vi "main.vi"() -> ()   [LabVIEW 2014]
doc: "This is the Main VI that uses Producer/Consumer Structure to present the UI.\nit consists of 2 taps for normal and admin users.\nadmin tab/interface is hidden by default until admin is logged in."
uses:
  <vilib>/addons/database/_DB Variant To Data/Database Variant To Data.xnode
panel:
  out "Cashier":dbl format="%#_6f"
  out "Logged User":string
  in  "Tab Control":enum32{"operator", "Supervisor"}(tab)
  in  "stop":bool
  in  "Purchase":bool
  in  "Quantity":dbl min=0.0
  in  "Product":string(combo)
  in  "Paid":dbl min=0.0 format="%#_6f"
  out "Cost":dbl format="%#_6f"
  out "Change":dbl format="%#_6f"
  in  "change user":bool
  in  "file name":path=path "C:/vendingMC/history.xml"
  in  "Time To":timestamp format="%<%H:%M:%S\n%Y/%m/%d>T"
  in  "Time From":timestamp format="%<%H:%M:%S\n%Y/%m/%d>T"
  in  "Price":dbl min=0.0
  in  "Type":string(combo)="normal"
  in  "Add Quantity":dbl
  in  "Generate XML":bool
  in  "add product":bool
  in  "Add Name":string
  in  "Delete User":bool
  in  "Register":bool
  in  "Edit password":string
  in  "Edit username":string
  # "Vending Machine"
  # "Select Product to Buy"
  # "Register New User"
  # "Add/Update Product"
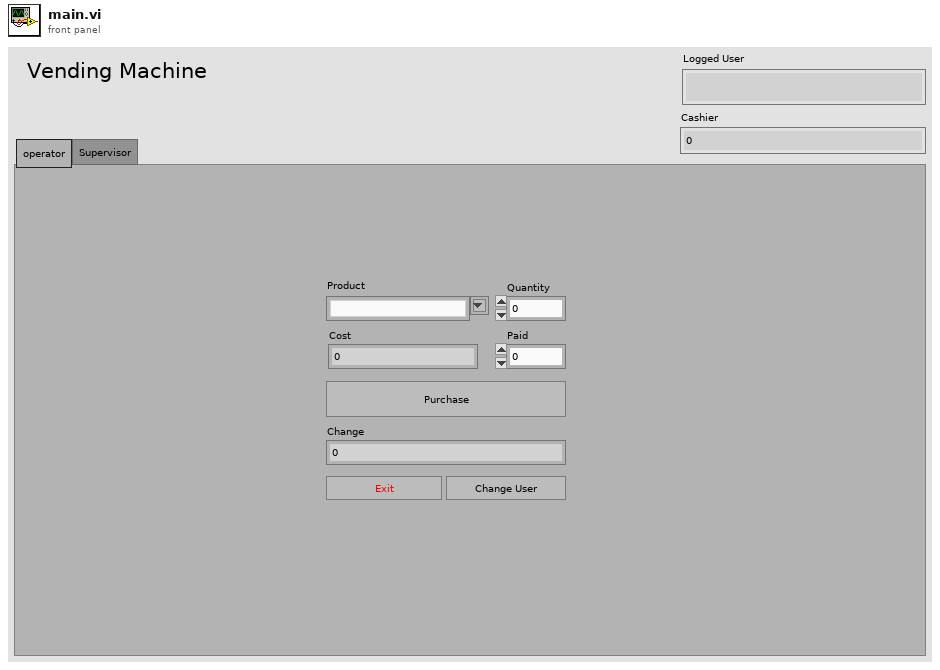
[diagram p1: front panel]
types:
  T1 = enum8{"Enabled", "Disabled", "Disabled and Grayed Out"}
  T2 = cluster{"date/time string":string, string, dbl, "Cost":dbl, dbl, dbl, "Logged User":string, "date/time string":string}
  T3 = enum16{"Left Button", "Center Button", "Right Button", "Window Close"}
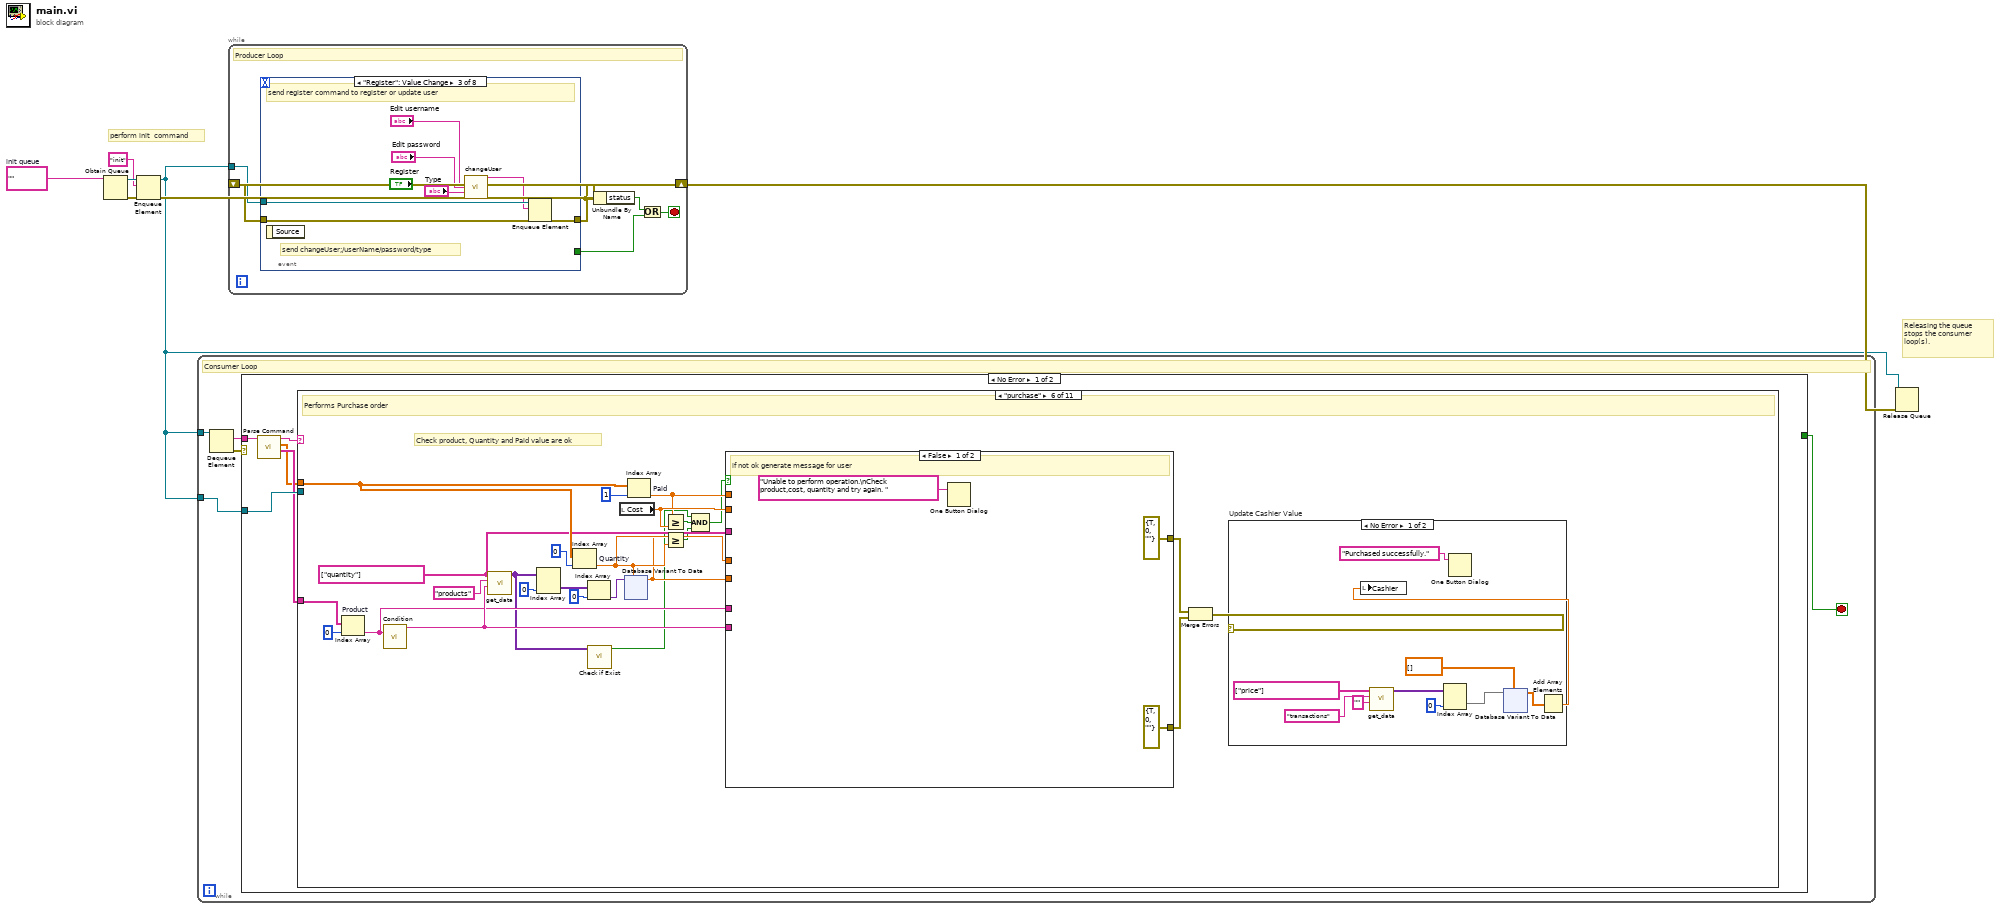
[diagram p0: block diagram]
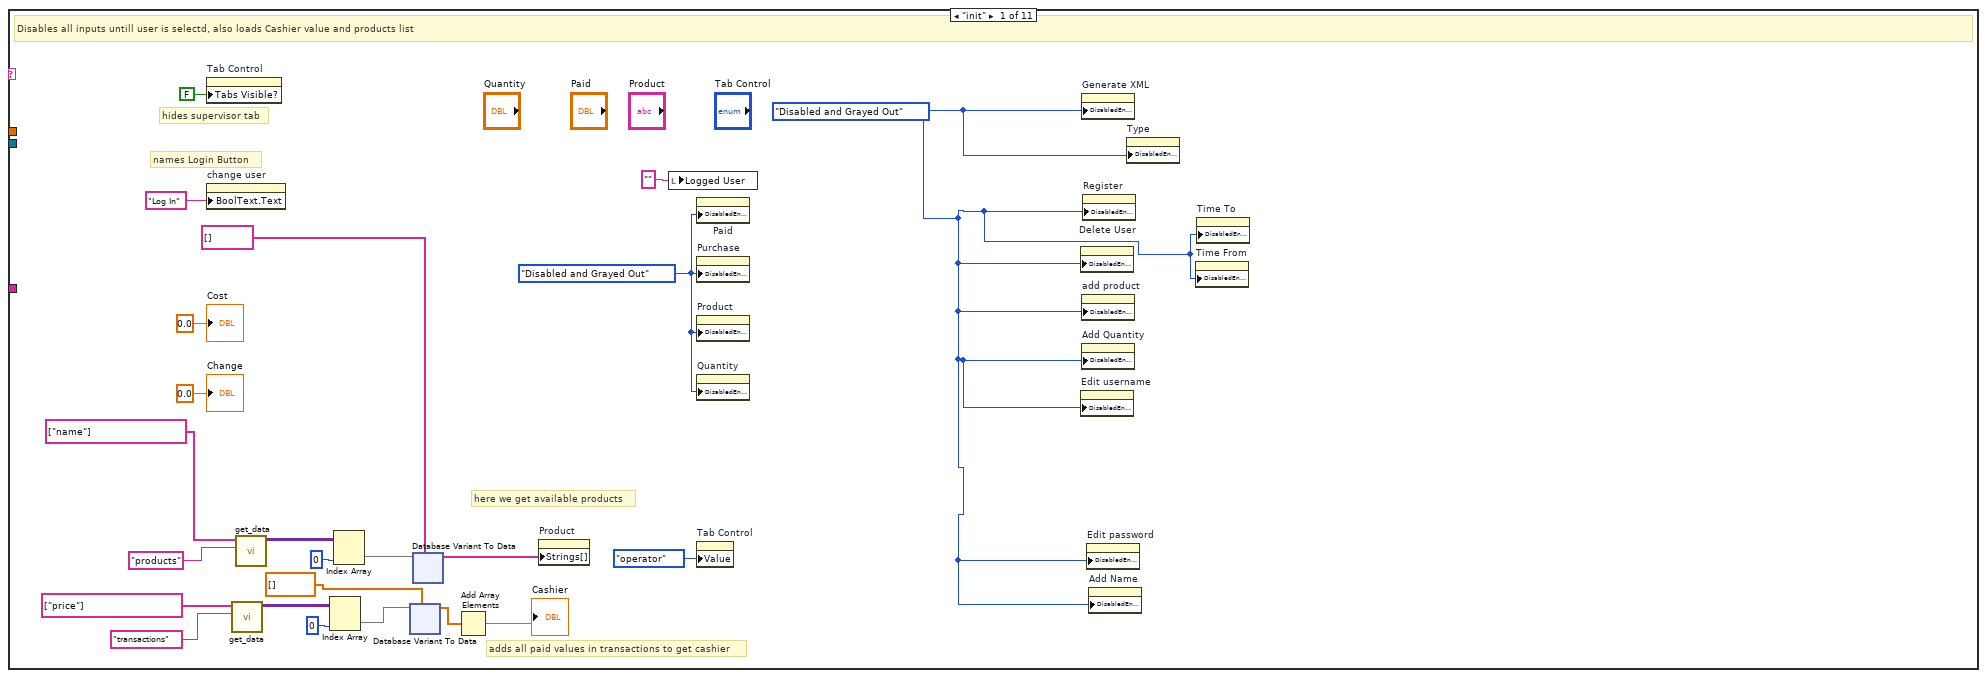
[diagram p2: hidden frame]
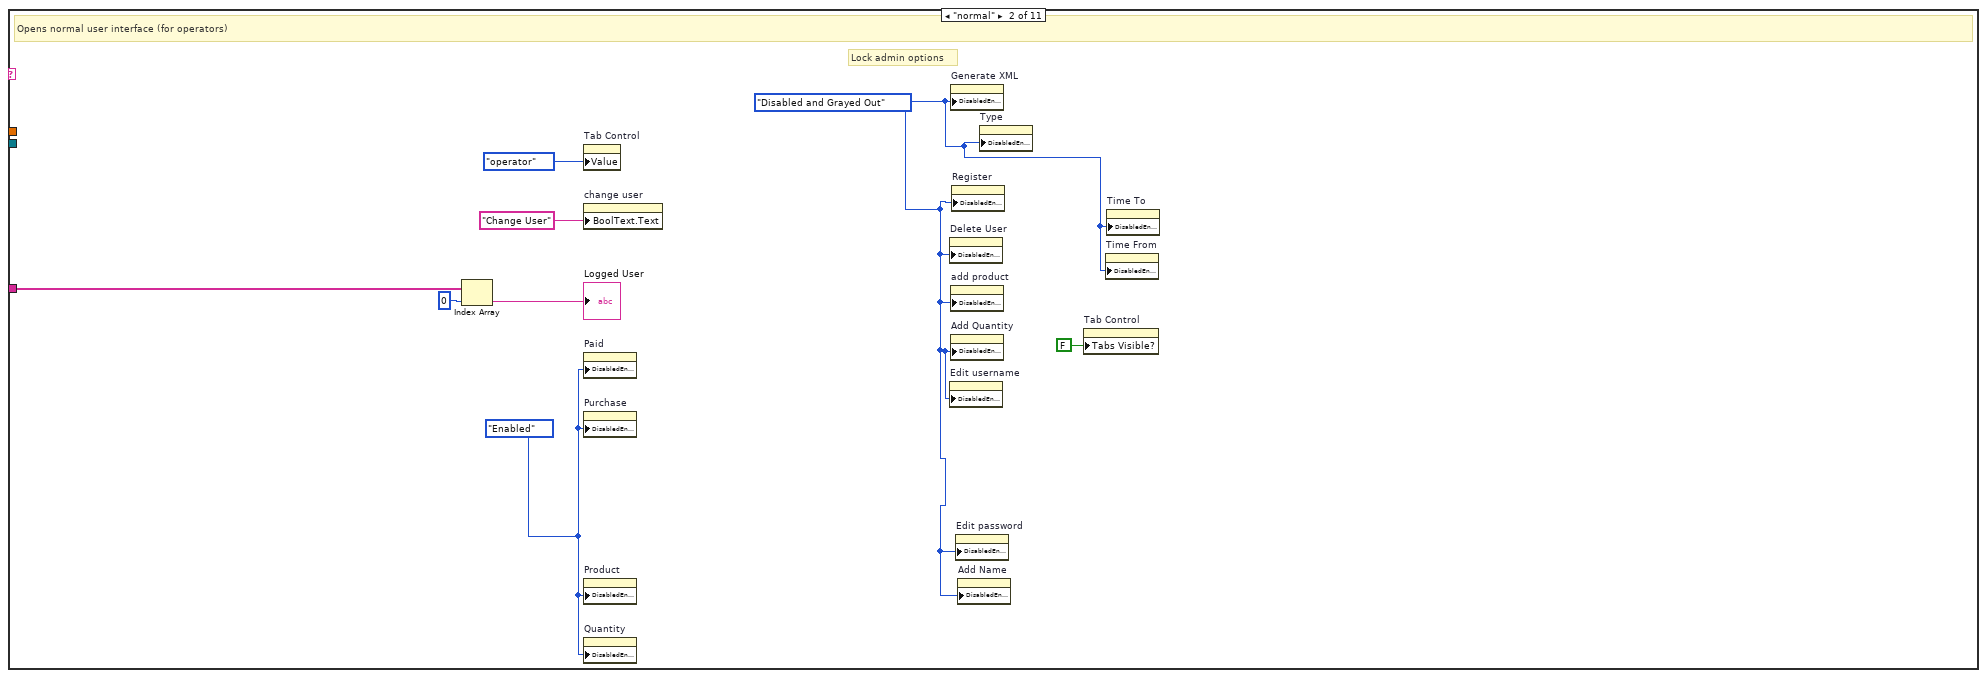
[diagram p3: hidden frame]
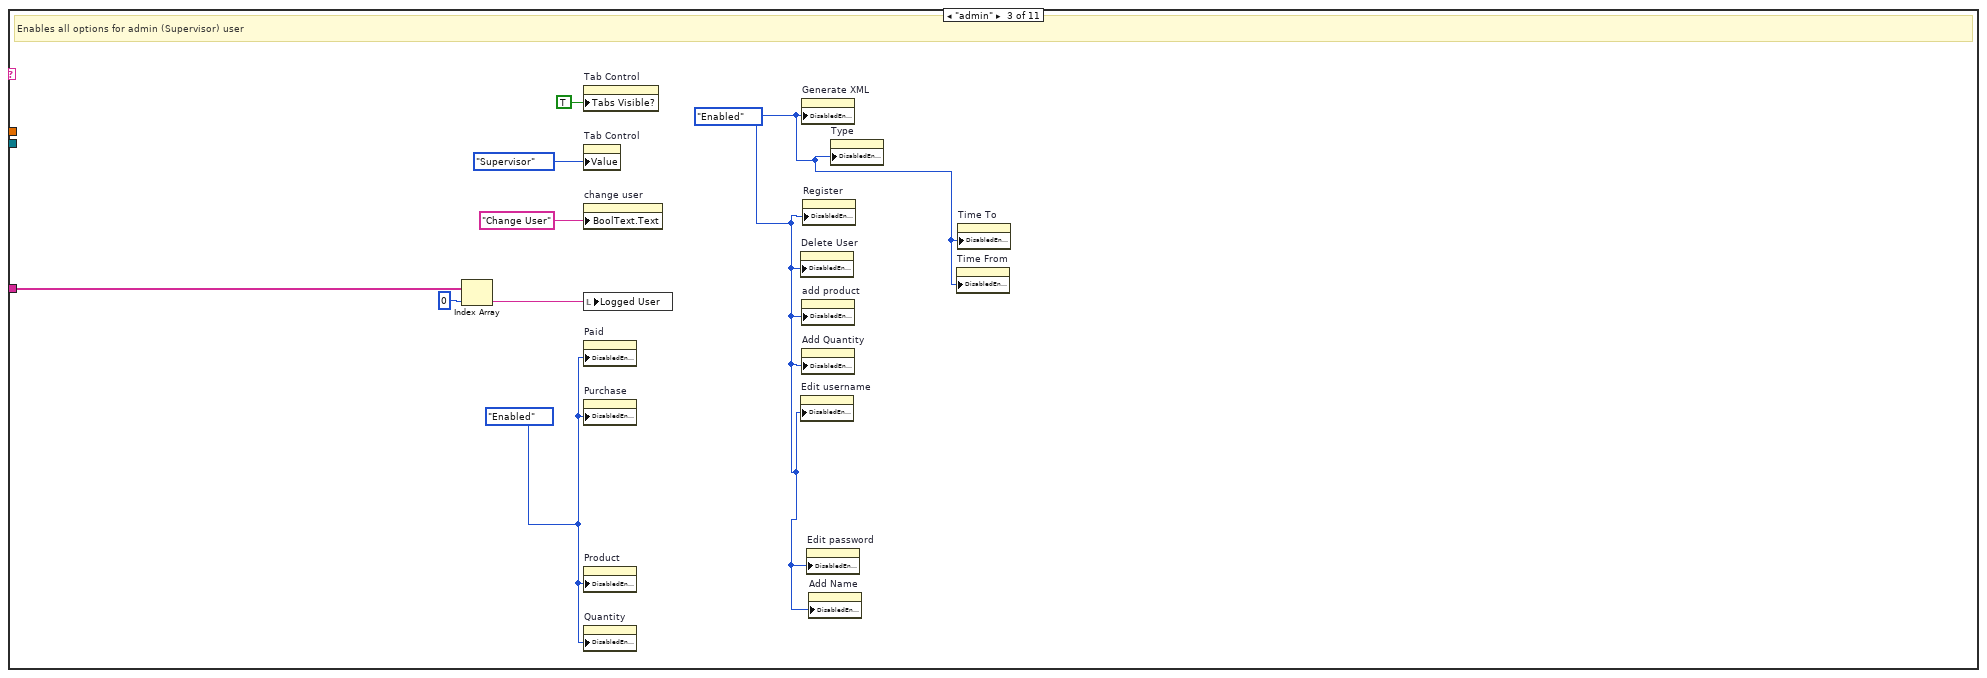
[diagram p4: hidden frame]
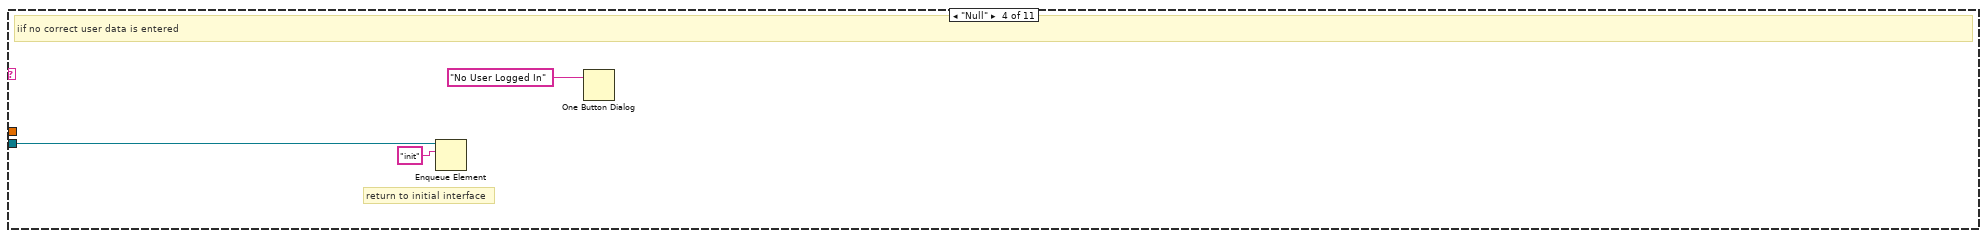
[diagram p5: hidden frame]
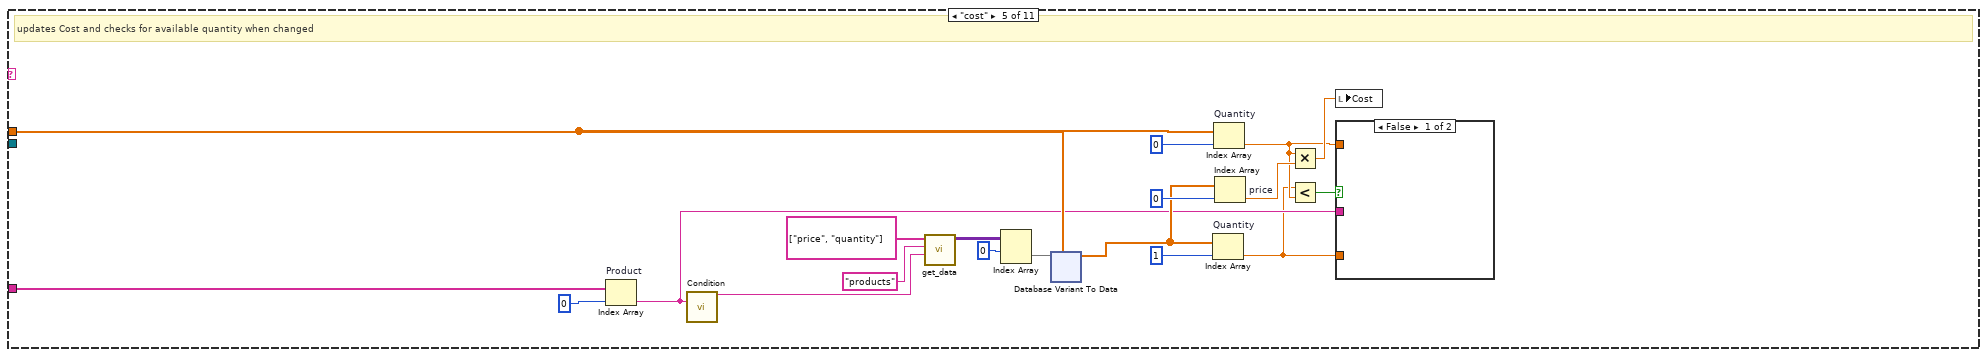
[diagram p6: hidden frame]
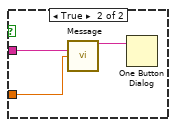
[diagram p7: hidden frame]
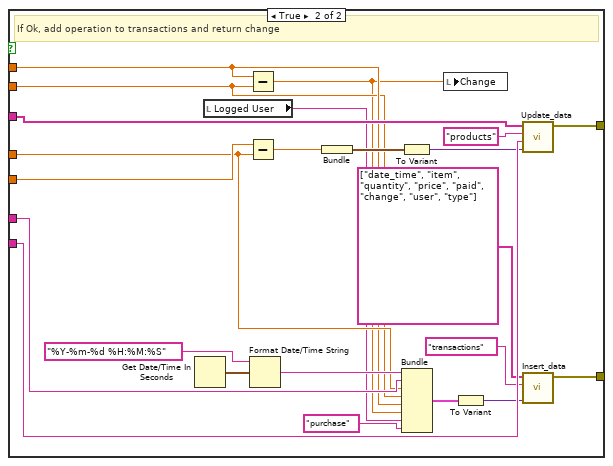
[diagram p9: hidden frame]
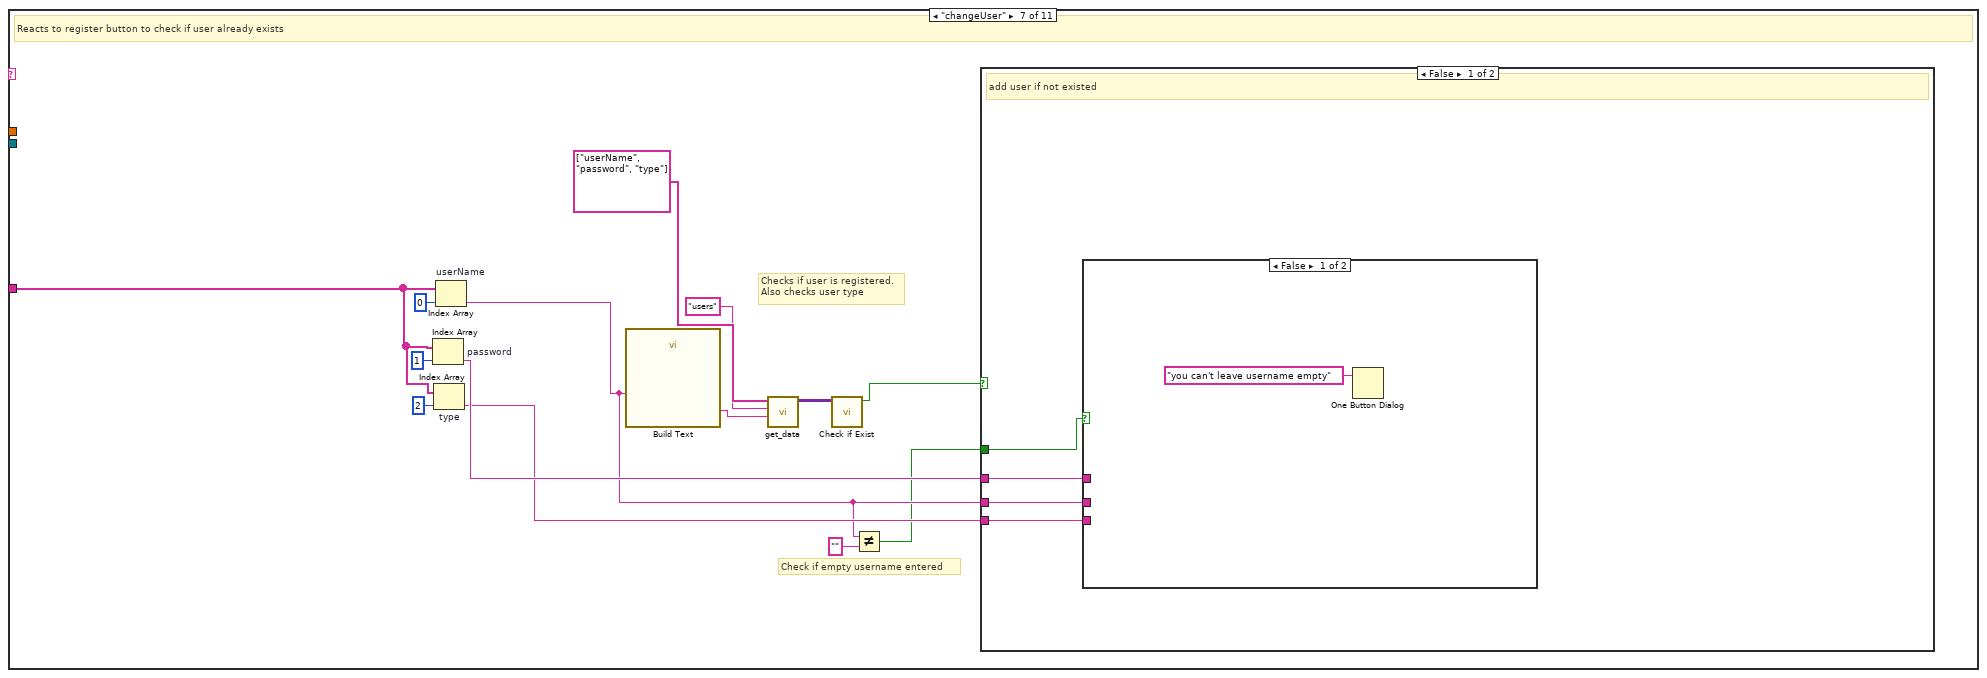
[diagram p10: hidden frame]
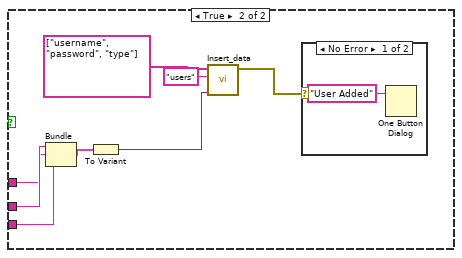
[diagram p11: hidden frame]
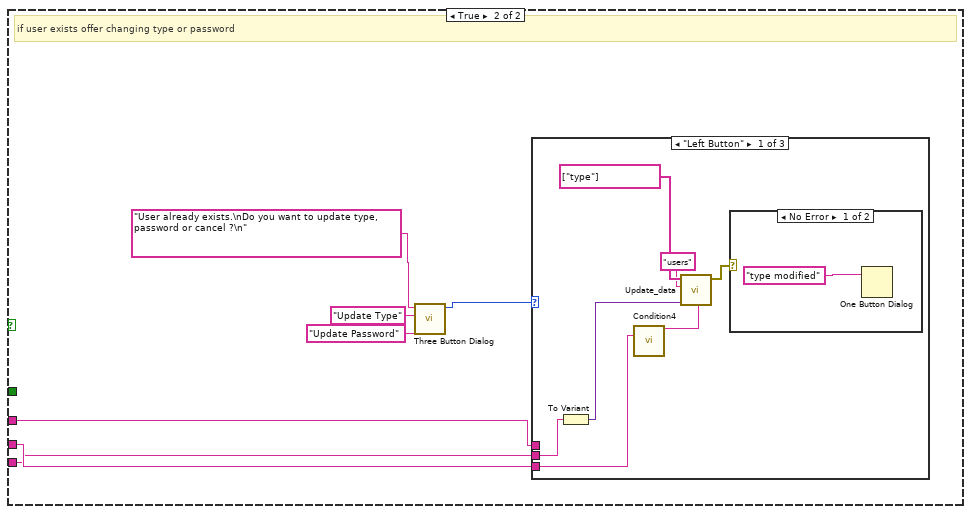
[diagram p13: hidden frame]
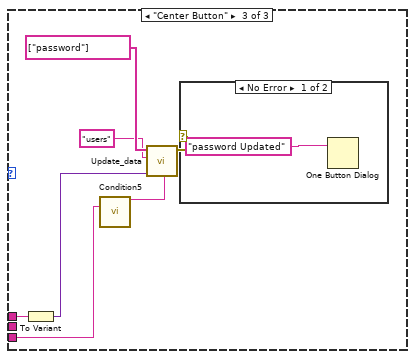
[diagram p16: hidden frame]
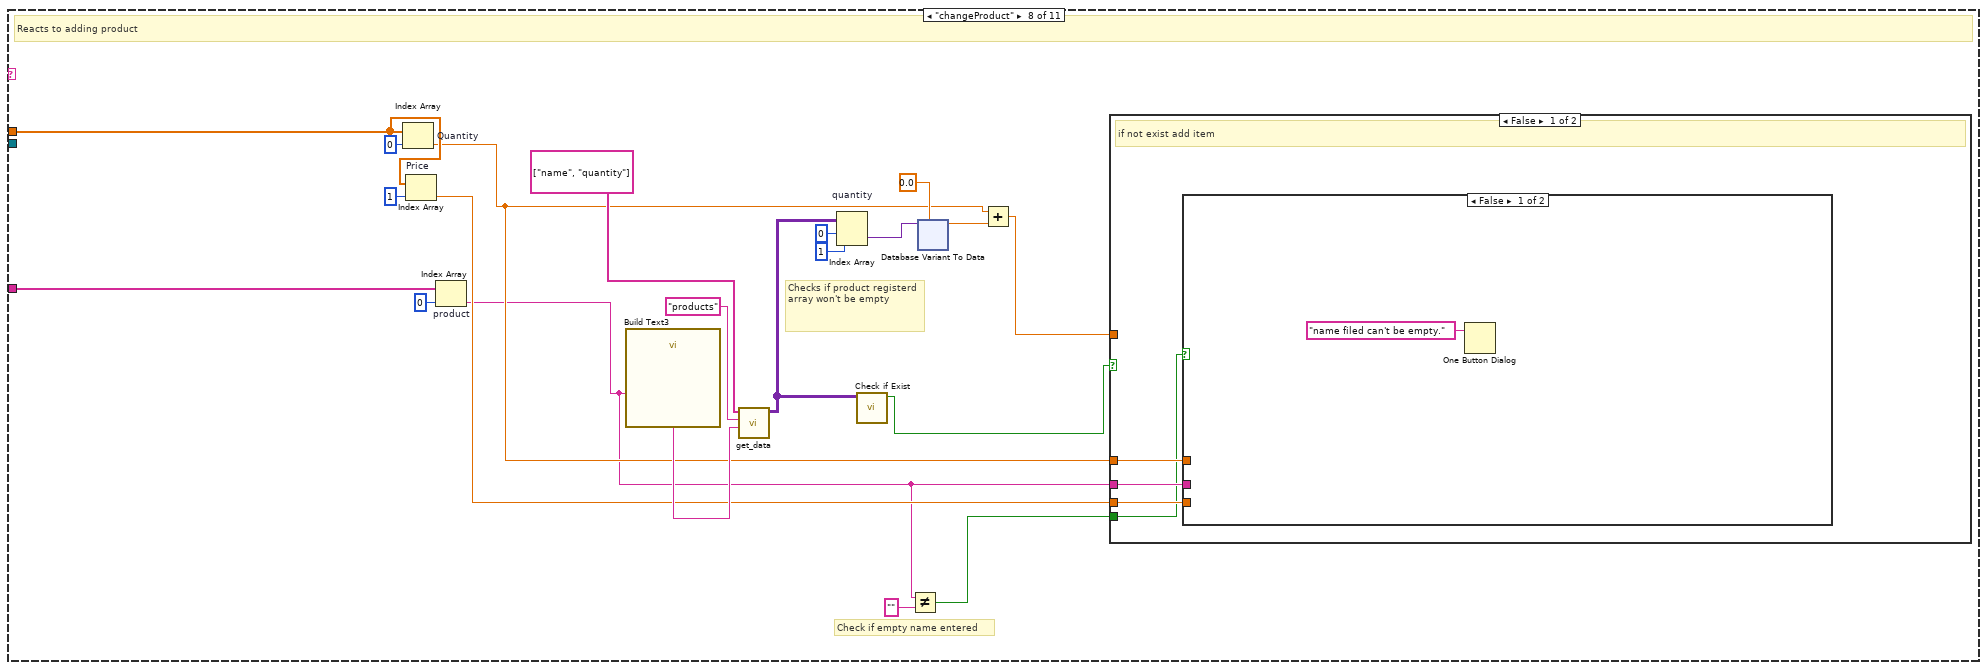
[diagram p18: hidden frame]
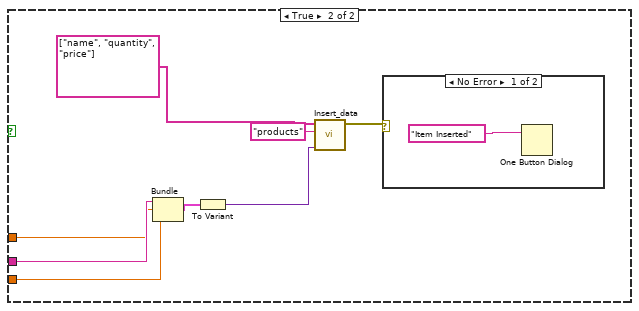
[diagram p19: hidden frame]
diagram:
  w6 = ""  # init queue
  # "perform init  command"
  # "Releasing the queue stops the consumer loop(s)."
  n1 = Obtain Queue(element data type=w6) -> (queue out=w5:refnum<queue>, error out=w3:errorcluster)  [unwired: 4 in, 1 out]
  n2 = Enqueue Element(queue=w5, element="init", error in (no error)=w3) -> (queue out=w1:refnum<queue>, error out=w4:errorcluster)  [unwired: 1 in, 1 out]
  n3 = while {
    tunnel: w1 -> [w12]
    tunnel: w1 -> [w8]
    stop <- w9 stop-if-true
    # "Consumer Loop"
    n4 = Dequeue Element(queue=w12) -> (element=w10:string, error out=w11:errorcluster)  [unwired: 2 in, 2 out]
    n5 = case shown="No Error" w11 {
      tunnel: w10 -> [w17 _]
      tunnel: [_ TRUE] -> w9
      tunnel: w8 -> [w15 _]
      frame No Error {
        n6 = call "Parse Command.vi"("command"=w17) -> ("Strings"=w14:string[], "numbers"=w13:dbl[], "Command"=w16:string)  [unwired: 8 in]
        n7 = case shown="\"purchase\"" w16 {
          tunnel: w15 -> [_ _ _ w134 _ _ _ _ _ _ _]
          tunnel: w14 -> [_ w124 w131 _ w154 w219 w333 w394 w473 w492 _]
          tunnel: w13 -> [_ _ _ _ w146 w220 _ w392 _ _ _]
          frame "init" {
            w18 = T1."Disabled and Grayed Out" ("Disabled")
            w39 = T1."Disabled and Grayed Out" ("Disabled")
            # "hides supervisor tab"
            # "names Login Button"
            # "adds all paid values in transactions to get cashier"
            # "here we get available products"
            # "Disables all inputs untill user is selectd, also loads Cashier value and products list"
            n8 = property on="Tab Control" class="TabCtl (strict)"("Tabs Visible?"=FALSE) -> ()  [unwired: 2 in, 2 out]
            n9 = property on="change user" class="Bool"("BoolText.Text"="Log In" ("Boolean Text.Text")) -> ()  [unwired: 2 in, 2 out]
            n10 = call "get_data.vi"("table"="transactions", "columns"=string[] ["price"]) -> ("Data"=w25:variant[][])  [unwired: 6 in, 3 out]
            n11 = call "get_data.vi"("table"="products", "columns"=string[] ["name"]) -> ("Data"=w32:variant[][])  [unwired: 6 in, 3 out]
            n12 = Index Array(array=w25, index (col)=0 ("index (row)")) -> (element=w23:variant[])  [unwired: 1 in]
            n13 = Index Array(array=w32, index (col)=0 ("index (row)")) -> (element=w35:variant[])  [unwired: 1 in]
            n14 = xnode "Database Variant To Data"("database variant"=w23, "type"=dbl[] [] ("numbers")) -> ("data"=w20:dbl[])  [unwired: 1 in, 1 out]
            n15 = xnode "Database Variant To Data"("database variant"=w35, "type"=string[] [] ("Strings []")) -> ("data"=w31:string[])  [unwired: 1 in, 1 out]
            n16 = Add Array Elements(numeric array=w20) -> (sum=→"Cashier":dbl)
            n17 = property on="Product" class="CmbBox"("Strings[]"=w31) -> ()  [unwired: 2 in, 2 out]
            n18 = local write "Logged User"("" ("Logged User")) -> ()
            n19 = property on="Paid" class="DigNum (strict)"("DisabledEnum"=w39) -> ()  [unwired: 2 in, 2 out]
            n20 = property on="Purchase" class="Bool"("DisabledEnum"=w39) -> ()  [unwired: 2 in, 2 out]
            n21 = property on="Product" class="CmbBox"("DisabledEnum"=w39) -> ()  [unwired: 2 in, 2 out]
            n22 = property on="Quantity" class="DigNum (strict)"("DisabledEnum"=w39) -> ()  [unwired: 2 in, 2 out]
            n23 = property on="Tab Control" class="TabCtl (strict)"("Value"=enum32{"operator", "Supervisor"}."operator" ("Tab Control")) -> ()  [unwired: 2 in, 2 out]
            n24 = property on="Delete User" class="Bool"("DisabledEnum"=w18) -> ()  [unwired: 2 in, 2 out]
            n25 = property on="Edit username" class="Str"("DisabledEnum"=w18) -> ()  [unwired: 2 in, 2 out]
            n26 = property on="Generate XML" class="Bool"("DisabledEnum"=w18) -> ()  [unwired: 2 in, 2 out]
            n27 = property on="add product" class="Bool"("DisabledEnum"=w18) -> ()  [unwired: 2 in, 2 out]
            n28 = property on="Add Quantity" class="DigNum (strict)"("DisabledEnum"=w18) -> ()  [unwired: 2 in, 2 out]
            n29 = property on="Register" class="Bool"("DisabledEnum"=w18) -> ()  [unwired: 2 in, 2 out]
            n30 = property on="Edit password" class="Str"("DisabledEnum"=w18) -> ()  [unwired: 2 in, 2 out]
            n31 = property on="Add Name" class="Str"("DisabledEnum"=w18) -> ()  [unwired: 2 in, 2 out]
            n32 = property on="Type" class="CmbBox"("DisabledEnum"=w18) -> ()  [unwired: 2 in, 2 out]
            n33 = property on="Time From" class="AbsTime (strict)"("DisabledEnum"=w18) -> ()  [unwired: 2 in, 2 out]
            n34 = property on="Time To" class="AbsTime (strict)"("DisabledEnum"=w18) -> ()  [unwired: 2 in, 2 out]
            "Cost" <- 0.0 ("Cost")
            "Change" <- 0.0 ("Change")
          }
          frame "normal" {
            w117 = T1."Disabled and Grayed Out" ("Disabled")
            w120 = T1."Enabled" ("Disabled")
            # "Lock admin options"
            # "Opens normal user interface (for operators)"
            n35 = Index Array(array=w124, index=0) -> (element=→"Logged User":string)
            n36 = property on="Tab Control" class="TabCtl (strict)"("Value"=enum32{"operator", "Supervisor"}."operator" ("Tab Control")) -> ()  [unwired: 2 in, 2 out]
            n37 = property on="change user" class="Bool"("BoolText.Text"="Change User" ("Boolean Text.Text")) -> ()  [unwired: 2 in, 2 out]
            n38 = property on="Paid" class="DigNum (strict)"("DisabledEnum"=w120) -> ()  [unwired: 2 in, 2 out]
            n39 = property on="Purchase" class="Bool"("DisabledEnum"=w120) -> ()  [unwired: 2 in, 2 out]
            n40 = property on="Product" class="CmbBox"("DisabledEnum"=w120) -> ()  [unwired: 2 in, 2 out]
            n41 = property on="Quantity" class="DigNum (strict)"("DisabledEnum"=w120) -> ()  [unwired: 2 in, 2 out]
            n42 = property on="Delete User" class="Bool"("DisabledEnum"=w117) -> ()  [unwired: 2 in, 2 out]
            n43 = property on="Edit username" class="Str"("DisabledEnum"=w117) -> ()  [unwired: 2 in, 2 out]
            n44 = property on="Generate XML" class="Bool"("DisabledEnum"=w117) -> ()  [unwired: 2 in, 2 out]
            n45 = property on="add product" class="Bool"("DisabledEnum"=w117) -> ()  [unwired: 2 in, 2 out]
            n46 = property on="Add Quantity" class="DigNum (strict)"("DisabledEnum"=w117) -> ()  [unwired: 2 in, 2 out]
            n47 = property on="Register" class="Bool"("DisabledEnum"=w117) -> ()  [unwired: 2 in, 2 out]
            n48 = property on="Edit password" class="Str"("DisabledEnum"=w117) -> ()  [unwired: 2 in, 2 out]
            n49 = property on="Add Name" class="Str"("DisabledEnum"=w117) -> ()  [unwired: 2 in, 2 out]
            n50 = property on="Type" class="CmbBox"("DisabledEnum"=w117) -> ()  [unwired: 2 in, 2 out]
            n51 = property on="Tab Control" class="TabCtl (strict)"("Tabs Visible?"=FALSE) -> ()  [unwired: 2 in, 2 out]
            n52 = property on="Time From" class="AbsTime (strict)"("DisabledEnum"=w117) -> ()  [unwired: 2 in, 2 out]
            n53 = property on="Time To" class="AbsTime (strict)"("DisabledEnum"=w117) -> ()  [unwired: 2 in, 2 out]
          }
          frame "admin" {
            w125 = T1."Enabled" ("Disabled")
            w128 = T1."Enabled" ("Disabled")
            # "Enables all options for admin (Supervisor) user"
            n54 = Index Array(array=w131, index=0) -> (element=w130:string)
            n55 = property on="Tab Control" class="TabCtl (strict)"("Tabs Visible?"=TRUE) -> ()  [unwired: 2 in, 2 out]
            n56 = property on="Tab Control" class="TabCtl (strict)"("Value"=enum32{"operator", "Supervisor"}."Supervisor" ("Tab Control")) -> ()  [unwired: 2 in, 2 out]
            n57 = property on="change user" class="Bool"("BoolText.Text"="Change User" ("Boolean Text.Text")) -> ()  [unwired: 2 in, 2 out]
            n58 = local write "Logged User"(w130) -> ()
            n59 = property on="Paid" class="DigNum (strict)"("DisabledEnum"=w128) -> ()  [unwired: 2 in, 2 out]
            n60 = property on="Purchase" class="Bool"("DisabledEnum"=w128) -> ()  [unwired: 2 in, 2 out]
            n61 = property on="Product" class="CmbBox"("DisabledEnum"=w128) -> ()  [unwired: 2 in, 2 out]
            n62 = property on="Quantity" class="DigNum (strict)"("DisabledEnum"=w128) -> ()  [unwired: 2 in, 2 out]
            n63 = property on="Delete User" class="Bool"("DisabledEnum"=w125) -> ()  [unwired: 2 in, 2 out]
            n64 = property on="Edit username" class="Str"("DisabledEnum"=w125) -> ()  [unwired: 2 in, 2 out]
            n65 = property on="Generate XML" class="Bool"("DisabledEnum"=w125) -> ()  [unwired: 2 in, 2 out]
            n66 = property on="add product" class="Bool"("DisabledEnum"=w125) -> ()  [unwired: 2 in, 2 out]
            n67 = property on="Add Quantity" class="DigNum (strict)"("DisabledEnum"=w125) -> ()  [unwired: 2 in, 2 out]
            n68 = property on="Register" class="Bool"("DisabledEnum"=w125) -> ()  [unwired: 2 in, 2 out]
            n69 = property on="Edit password" class="Str"("DisabledEnum"=w125) -> ()  [unwired: 2 in, 2 out]
            n70 = property on="Add Name" class="Str"("DisabledEnum"=w125) -> ()  [unwired: 2 in, 2 out]
            n71 = property on="Type" class="CmbBox"("DisabledEnum"=w125) -> ()  [unwired: 2 in, 2 out]
            n72 = property on="Time From" class="AbsTime (strict)"("DisabledEnum"=w125) -> ()  [unwired: 2 in, 2 out]
            n73 = property on="Time To" class="AbsTime (strict)"("DisabledEnum"=w125) -> ()  [unwired: 2 in, 2 out]
          }
          frame "Null" {
            # "return to initial interface"
            # "iif no correct user data is entered"
            n74 = Enqueue Element(queue=w134, element="init") -> ()  [unwired: 2 in, 3 out]
            n75 = One Button Dialog(message="No User Logged In") -> ()  [unwired: 1 in, 1 out]
          }
          frame "cost" {
            # "updates Cost and checks for available quantity when changed"
            n76 = Index Array "Product"(array=w154, index=0) -> (element=w139:string)
            n77 = call "Condition"("name"=w139) -> ("Result"=w149:string)  [unwired: 13 in, 1 out]
            n78 = call "get_data.vi"("condition"=w149, "table"="products", "columns"=string[] ["price", "quantity"]) -> ("Data"=w148:variant[][])  [unwired: 5 in, 3 out]
            n79 = Index Array(array=w148, index (row)=0 ("disabled index (col)")) -> (element=w147:variant[])  [unwired: 1 in]
            n80 = xnode "Database Variant To Data"("database variant"=w147, "type"=w146) -> ("data"=w142:dbl[])  [unwired: 1 in, 1 out]
            n81 = Index Array "Quantity"(array=w142, index=1) -> (element=w136:dbl)
            n82 = Index Array "Quantity"(array=w146, index=0) -> (element=w138:dbl)
            n83 = Index Array "price"(array=w142, index=0) -> (element=w144:dbl)
            n84 = Multiply(x=w138, y=w144) -> (x*y=w143:dbl)
            n85 = Less?(x=w136, y=w138) -> (x < y?=w140:bool)
            n86 = local write "Cost"(w143) -> ()
            n87 = case shown="False" w140 {
              tunnel: w139 -> [_ w157]
              tunnel: w138 -> [_ _]
              tunnel: w136 -> [_ w155]
              frame False {
              }
              frame True {
                n88 = call "Message"("product"=w157, "max"=w155) -> ("Result"=w156:string)  [unwired: 12 in, 1 out]
                n89 = One Button Dialog(message=w156) -> ()  [unwired: 1 in, 1 out]
              }
            }
          }
          frame "purchase" {
            w209 = string[] ["quantity"] ("columns")
            # "Check product, Quantity and Paid value are ok"
            # "Performs Purchase order"
            n90 = Index Array "Product"(array=w219, index=0) -> (element=w206:string)
            n91 = call "Condition"("name"=w206) -> ("Result"=w210:string)  [unwired: 13 in, 1 out]
            n92 = call "get_data.vi"("condition"=w210, "table"="products", "columns"=w209) -> ("Data"=w200:variant[][])  [unwired: 5 in, 3 out]
            n93 = Index Array(array=w200, index (col)=0 ("index (row)")) -> (element=w213:variant[])  [unwired: 1 in]
            n94 = Index Array "Quantity"(array=w220, index=0) -> (element=w208:dbl)
            n95 = Index Array(array=w213, index=0) -> (element=w211:variant)
            n96 = call "Check if Exist.vi"("Data"=w200) -> ("Boolean"=w199:bool)  [unwired: 10 in]
            n97 = local read "Cost"() -> (w205:dbl)
            n98 = xnode "Database Variant To Data"("database variant"=w211, "type"=w208) -> ("data"=w207:dbl)  [unwired: 1 in, 1 out]
            n99 = Index Array "Paid"(array=w220, index=1) -> (element=w204:dbl)
            n100 = Greater Or Equal?(x=w204, y=w205) -> (x >= y?=w198:bool)
            n101 = Greater Or Equal?(x=w207, y=w208) -> (x >= y?=w197:bool)
            n102 = Compound Arithmetic op=AND(w199, w198, w197) -> (w196:bool)
            n103 = case shown="False" w196 {
              tunnel: w210 -> [_ w293]
              tunnel: w209 -> [_ w292]
              tunnel: w208 -> [_ w281]
              tunnel: w207 -> [_ w288]
              tunnel: w206 -> [_ w282]
              tunnel: w205 -> [_ w279]
              tunnel: w204 -> [_ w280]
              tunnel: [errorcluster {"status"=TRUE, "code"=0, "source"=""} ("error out") w273] -> w202
              tunnel: [errorcluster {"status"=TRUE, "code"=0, "source"=""} ("error out") w272] -> w203
              frame False {
                # "if not ok generate message for user"
                n104 = One Button Dialog(message="Unable to perform operation.\nCheck product,cost, quantity and try again. ") -> ()  [unwired: 1 in, 1 out]
              }
              frame True {
                # "If Ok, add operation to transactions and return change"
                n105 = Get Date/Time In Seconds() -> (seconds since 1Jan1904=w286:timestamp)
                n106 = local read "Logged User"() -> (w277:string)
                n107 = Subtract(x=w280, y=w279) -> (x-y=w274:dbl)
                n108 = Subtract(x=w288, y=w281) -> (x-y=w290:dbl)
                n109 = Format Date/Time String(time format string (%c)="%Y-%m-%d %H:%M:%S", seconds (now)=w286) -> (date/time string=w283:string)  [unwired: 1 in]
                n110 = Bundle(w290) -> (w291:cluster{dbl})  [unwired: 1 in]
                n111 = To Variant(anything=w291) -> (Variant=w289:variant)
                n112 = Bundle("date/time string"=w283, w282, w281, "Cost"=w279, w280, w274, "Logged User"=w277, "date/time string"="purchase") -> (w276:T2)  [unwired: 1 in]
                n113 = local write "Change"(w274) -> ()
                n114 = To Variant(anything=w276) -> (Variant=w275:variant)
                n115 = call "Update_data.vi"("input data"=w289, "condition"=w293, "table"="products", "columns"=w292) -> ("error out"=w272:errorcluster)  [unwired: 4 in, 3 out]
                n116 = call "Insert_data.vi"("input data"=w275, "table"="transactions", "columns"=string[] ["date_time", "item", "quantity", "price", "paid", "change", "user", "type"]) -> ("error out"=w273:errorcluster)  [unwired: 5 in, 3 out]
              }
            }
            n117 = Merge Errors(w203, w202) -> (w201:errorcluster)
            n118 = case "Update Cashier Value" shown="No Error" w201 {
              frame No Error {
                n119 = call "get_data.vi"("condition"="", "table"="transactions", "columns"=string[] ["price"]) -> ("Data"=w228:variant[][])  [unwired: 5 in, 3 out]
                n120 = Index Array(array=w228, index (col)=0 ("index (row)")) -> (element=w226:variant[])  [unwired: 1 in]
                n121 = One Button Dialog(message="Purchased successfully.") -> ()  [unwired: 1 in, 1 out]
                n122 = xnode "Database Variant To Data"("database variant"=w226, "type"=dbl[] [] ("numbers")) -> ("data"=w224:dbl[])  [unwired: 1 in, 1 out]
                n123 = Add Array Elements(numeric array=w224) -> (sum=w222:dbl)
                n124 = local write "Cashier"(w222) -> ()
              }
              frame Error {
              }
            }
          }
          frame "changeUser" {
            # "Check if empty username entered"
            # "Checks if user is registered.\nAlso checks user type"
            # "Reacts to register button to check if user already exists"
            n125 = Index Array "password"(array=w333, index=1) -> (element=w332:string)
            n126 = Index Array "type"(array=w333, index=2) -> (element=w331:string)
            n127 = Index Array "userName"(array=w333, index=0) -> (element=w330:string)
            n128 = call "Build Text"("username"=w330) -> ("Result"=w338:string)  [unwired: 13 in, 1 out]
            n129 = call "get_data.vi"("condition"=w338, "table"="users", "columns"=string[] ["userName", "password", "type"]) -> ("Data"=w337:variant[][])  [unwired: 5 in, 3 out]
            n130 = call "Check if Exist.vi"("Data"=w337) -> ("Boolean"=w328:bool)  [unwired: 10 in]
            n131 = Not Equal?(x=w330, y="") -> (x != y?=w327:bool)
            n132 = case shown="False" w328 {
              tunnel: w330 -> [w344 w357]
              tunnel: w332 -> [w343 w356]
              tunnel: w331 -> [w342 w355]
              tunnel: w327 -> [w341 _]
              frame False {
                # "add user if not existed"
                n133 = case shown="False" w341 {
                  tunnel: w344 -> [_ w349]
                  tunnel: w343 -> [_ w348]
                  tunnel: w342 -> [_ w347]
                  frame False {
                    n134 = One Button Dialog(message="you can't leave username empty") -> ()  [unwired: 1 in, 1 out]
                  }
                  frame True {
                    n135 = Bundle(w349, w348, w347) -> (w351:cluster{string, string, string})  [unwired: 1 in]
                    n136 = To Variant(anything=w351) -> (Variant=w350:variant)
                    n137 = call "Insert_data.vi"("input data"=w350, "table"="users", "columns"=string[] ["username", "password", "type"]) -> ("error out"=w346:errorcluster)  [unwired: 5 in, 3 out]
                    n138 = case shown="No Error" w346 {
                      frame No Error {
                        n139 = One Button Dialog(message="User Added") -> ()  [unwired: 1 in, 1 out]
                      }
                      frame Error {
                      }
                    }
                  }
                }
              }
              frame True {
                # "if user exists offer changing type or password"
                n140 = call <vilib>:"Three Button Dialog.vi"("Center Button Text (\"No\")"="Update Password" ("Center Button Text (\"No\")"), "Left Button Text (\"Yes\")"="Update Type" ("Left Button Text (\"Yes\")"), "message"="User already exists.\nDo you want to update type, password or cancel ?\n") -> ("Which Button?"=w358:T3)  [unwired: 8 in]
                n141 = case shown="\"Left Button\"" w358 {
                  tunnel: w357 -> [w364 _ w373]
                  tunnel: w356 -> [_ _ w370]
                  tunnel: w355 -> [w362 _ _]
                  frame "Left Button" {
                    n142 = To Variant(anything=w362) -> (Variant=w363:variant)
                    n143 = call "Condition4"("name"=w364) -> ("Result"=w366:string)  [unwired: 13 in, 1 out]
                    n144 = call "Update_data.vi"("input data"=w363, "condition"=w366, "table"="users", "columns"=string[] ["type"]) -> ("error out"=w365:errorcluster)  [unwired: 4 in, 3 out]
                    n145 = case shown="No Error" w365 {
                      frame No Error {
                        n146 = One Button Dialog(message="type modified") -> ()  [unwired: 1 in, 1 out]
                      }
                      frame Error {
                      }
                    }
                  }
                  frame "Right Button", Default {
                  }
                  frame "Center Button" {
                    n147 = To Variant(anything=w370) -> (Variant=w371:variant)
                    n148 = call "Condition5"("name"=w373) -> ("Result"=w374:string)  [unwired: 13 in, 1 out]
                    n149 = call "Update_data.vi"("input data"=w371, "condition"=w374, "table"="users", "columns"=string[] ["password"]) -> ("error out"=w372:errorcluster)  [unwired: 4 in, 3 out]
                    n150 = case shown="No Error" w372 {
                      frame No Error {
                        n151 = One Button Dialog(message="password Updated") -> ()  [unwired: 1 in, 1 out]
                      }
                      frame Error {
                      }
                    }
                  }
                }
              }
            }
          }
          frame "changeProduct" {
            # "Check if empty name entered"
            # "Checks if product registerd array won't be empty"
            # "Reacts to adding product"
            n152 = Index Array "Quantity"(array=w392, index=0) -> (element=w384:dbl)
            n153 = Index Array "Price"(array=w392, index=1) -> (element=w390:dbl)
            n154 = Index Array "product"(array=w394, index=0) -> (element=w378:string)
            n155 = call "Build Text3"("name"=w378) -> ("Result"=w396:string)  [unwired: 13 in, 1 out]
            n156 = call "get_data.vi"("condition"=w396, "table"="products", "columns"=string[] ["name", "quantity"]) -> ("Data"=w381:variant[][])  [unwired: 5 in, 3 out]
            n157 = Index Array "quantity"(array=w381, index (row)=0, index (col)=1 ("disabled index (col)")) -> (element=w387:variant)
            n158 = call "Check if Exist.vi"("Data"=w381) -> ("Boolean"=w382:bool)  [unwired: 10 in]
            n159 = Not Equal?(x=w378, y="") -> (x != y?=w379:bool)
            n160 = xnode "Database Variant To Data"("database variant"=w387, "type"=0.0 ("element")) -> ("data"=w385:dbl)  [unwired: 1 in, 1 out]
            n161 = Add(x=w384, y=w385) -> (x+y=w383:dbl)
            n162 = case shown="False" w382 {
              tunnel: w378 -> [w434 w451]
              tunnel: w384 -> [w433 _]
              tunnel: w390 -> [w432 w445]
              tunnel: w383 -> [_ w446]
              tunnel: w379 -> [w431 _]
              frame False {
                # "if not exist add item"
                n163 = case shown="False" w431 {
                  tunnel: w434 -> [_ w440]
                  tunnel: w433 -> [_ w439]
                  tunnel: w432 -> [_ w438]
                  frame False {
                    n164 = One Button Dialog(message="name filed can't be empty.") -> ()  [unwired: 1 in, 1 out]
                  }
                  frame True {
                    n165 = Bundle(w440, w439, w438) -> (w442:cluster{string, dbl, dbl})  [unwired: 1 in]
                    n166 = To Variant(anything=w442) -> (Variant=w441:variant)
                    n167 = call "Insert_data.vi"("input data"=w441, "table"="products", "columns"=string[] ["name", "quantity", "price"]) -> ("error out"=w436:errorcluster)  [unwired: 5 in, 3 out]
                    n168 = case shown="No Error" w436 {
                      frame No Error {
                        n169 = One Button Dialog(message="Item Inserted") -> ()  [unwired: 1 in, 1 out]
                      }
                      frame Error {
                      }
                    }
                  }
                }
              }
              frame True {
                # "if exist offer adding quantity or updating product price"
                n170 = call <vilib>:"Three Button Dialog.vi"("Center Button Text (\"No\")"="Update Price" ("Center Button Text (\"No\")"), "Left Button Text (\"Yes\")"="Add to Quantity" ("Left Button Text (\"Yes\")"), "message"="Product already exists.\nDo you want to update Quantity, price or cancel ?\n") -> ("Which Button?"=w447:T3)  [unwired: 8 in]
                n171 = case shown="\"Left Button\"" w447 {
                  tunnel: w451 -> [w454 _ w463]
                  tunnel: w446 -> [w452 _ _]
                  tunnel: w445 -> [_ _ w460]
                  frame "Left Button" {
                    # "add quantity"
                    n172 = To Variant(anything=w452) -> (Variant=w453:variant)
                    n173 = call "Condition3"("name"=w454) -> ("Result"=w456:string)  [unwired: 13 in, 1 out]
                    n174 = call "Update_data.vi"("input data"=w453, "condition"=w456, "table"="products", "columns"=string[] ["Quantity"]) -> ("error out"=w455:errorcluster)  [unwired: 4 in, 3 out]
                    n175 = case shown="No Error" w455 {
                      frame No Error {
                        n176 = One Button Dialog(message="Quantity added") -> ()  [unwired: 1 in, 1 out]
                      }
                      frame Error {
                      }
                    }
                  }
                  frame "Right Button", Default {
                  }
                  frame "Center Button" {
                    # "change price"
                    n177 = To Variant(anything=w460) -> (Variant=w461:variant)
                    n178 = call "Condition2"("name"=w463) -> ("Result"=w464:string)  [unwired: 13 in, 1 out]
                    n179 = call "Update_data.vi"("input data"=w461, "condition"=w464, "table"="products", "columns"=string[] ["price"]) -> ("error out"=w462:errorcluster)  [unwired: 4 in, 3 out]
                    n180 = case shown="No Error" w462 {
                      frame No Error {
                        n181 = One Button Dialog(message="Price Updated") -> ()  [unwired: 1 in, 1 out]
                      }
                      frame Error {
                      }
                    }
                  }
                }
              }
            }
          }
          frame "deleteUser" {
            # "Checks if user is registered.\nAlso checks user type"
            # "delete existing user"
            n182 = Index Array "password"(array=w473, index=1) -> (element=w471:string)
            n183 = Index Array "type"(array=w473, index=2) -> (element=w470:string)
            n184 = Index Array "userName"(array=w473, index=0) -> (element=w472:string)
            n185 = call "Build Text2"("username"=w472) -> ("Result"=w477:string)  [unwired: 13 in, 1 out]
            n186 = call "get_data.vi"("condition"=w477, "table"="users", "columns"=string[] ["userName", "password", "type"]) -> ("Data"=w469:variant[][])  [unwired: 5 in, 3 out]
            n187 = call "Check if Exist.vi"("Data"=w469) -> ("Boolean"=w468:bool)  [unwired: 10 in]
            n188 = case shown="False" w468 {
              tunnel: w472 -> [_ w482]
              tunnel: w471 -> [_ _]
              tunnel: w470 -> [_ _]
              frame False {
                # "user don't exist"
                n189 = One Button Dialog(message="User don't exists.\n") -> ()  [unwired: 1 in, 1 out]
              }
              frame True {
                # "Delete user"
                n190 = call "Condition"("name"=w482) -> ("Result"=w483:string)  [unwired: 13 in, 1 out]
                n191 = call "delete_data.vi"("table"="users", "condition"=w483) -> ("error out"=w481:errorcluster)  [unwired: 6 in, 3 out]
                n192 = case shown="No Error" w481 {
                  frame No Error {
                    n193 = One Button Dialog(message="User deleted\n") -> ()  [unwired: 1 in, 1 out]
                  }
                  frame Error {
                  }
                }
              }
            }
          }
          frame "generateXML" {
            # "Generate XML data at chosen file for transactions at time/date selected"
            n194 = Index Array "date from"(array=w492, index=0) -> (element=w488:string)
            n195 = Index Array "date to"(array=w492, index=1) -> (element=w487:string)
            n196 = call "GenXML.vi"("dateTo"=w487, "dateFrom"=w488, "file name"="file name") -> ("error out"=w486:errorcluster)  [unwired: 6 in, 2 out]
            n197 = case shown="No Error" w486 {
              frame No Error {
                n198 = One Button Dialog(message="File Generated successfully.") -> ()  [unwired: 1 in, 1 out]
              }
              frame Error {
              }
            }
          }
          frame Default {
            # "default, do nothing"
          }
        }
      }
      frame Error {
        # "Return true in any case that should stop the loop."
      }
    }
  }
  n199 = while {
    shift-right: [w496] -> w7
    shift-left: w4 -> [w499]
    tunnel: w1 -> [w500]
    stop <- w497 stop-if-true
    # "Producer Loop"
    n200 = event shown="[2] \"Register\": Value Change" {
      selector: _ -> [_ _ _ _ _ _ _ _]
      dyn-events: _ -> [_ _ _ _ _ _ _ _]
      timeout: _ -> [_ _ _ _ _ _ _ _]
      tunnel: w500 -> [w507 w513 w520 w527 w536 w543 w549 _]
      tunnel: w499 -> [w506 w512 w519 w526 w535 w542 w548 w550]
      tunnel: [w505 w511 w518 w525 w534 w541 w547 w550] -> w496
      tunnel: [_ _ _ _ _ _ _ "stop"] -> w498
      event "Purchase": Value Change {
        # "send purchase;quantity,paid/product"
        # "Sends purchase command"
        n201 = event-data() -> ()  [unwired: 1 in, 1 out]
        n202 = local read "Quantity"() -> (w503:dbl)
        n203 = local read "Product"() -> (w501:string)
        n204 = local read "Paid"() -> (w502:dbl)
        n205 = call "Purchase"("quantity"=w503, "paid"=w502, "product"=w501) -> ("Result"=w504:string)  [unwired: 11 in, 1 out]
        n206 = Enqueue Element(queue=w507, element=w504, error in (no error)=w506) -> (error out=w505:errorcluster)  [unwired: 1 in, 2 out]
      }
      event "change user": Value Change {
        # "send userType;/userName"
        # "Check for credentials and identifies user"
        n207 = event-data() -> ()  [unwired: 1 in, 1 out]
        n208 = call "Log In.vi"() -> ("user type"=w509:string, "username"=w508:string)  [unwired: 9 in, 1 out]
        n209 = call "logIn"("userType"=w509, "userName"=w508) -> ("Result"=w510:string)  [unwired: 12 in, 1 out]
        n210 = Enqueue Element(queue=w513, element=w510, error in (no error)=w512) -> (error out=w511:errorcluster)  [unwired: 1 in, 2 out]
      }
      event "Register": Value Change {
        # "send changeUser;/userName/password/type"
        # "send register command to register or update user"
        n211 = event-data() -> ()  [unwired: 1 in, 1 out]
        n212 = call "changeUser"("userName"="Edit username", "password"="Edit password", "type"="Type") -> ("Result"=w517:string)  [unwired: 11 in, 1 out]
        n213 = Enqueue Element(queue=w520, element=w517, error in (no error)=w519) -> (error out=w518:errorcluster)  [unwired: 1 in, 2 out]
      }
      event "add product": Value Change {
        # "send changeProduct;quantity,price/product"
        # "Sends changeProduct command"
        n214 = event-data() -> ()  [unwired: 1 in, 1 out]
        n215 = call "changeProduct"("quantity"="Add Quantity", "price"="Price", "product"="Add Name") -> ("Result"=w524:string)  [unwired: 11 in, 1 out]
        n216 = Enqueue Element(queue=w527, element=w524, error in (no error)=w526) -> (error out=w525:errorcluster)  [unwired: 1 in, 2 out]
      }
      event "Generate XML": Value Change {
        w530 = "%Y-%m-%d %H:%M:%S" ("time format string (%c)")
        # "send generateXML;/timeFrom/timeTo"
        # "Generate XML File"
        n217 = event-data() -> ()  [unwired: 1 in, 1 out]
        n218 = Format Date/Time String(time format string (%c)=w530, seconds (now)="Time From") -> (date/time string=w529:string)  [unwired: 1 in]
        n219 = Format Date/Time String(time format string (%c)=w530, seconds (now)="Time To") -> (date/time string=w528:string)  [unwired: 1 in]
        n220 = call "generateXML"("timeFrom"=w529, "timeTo"=w528) -> ("Result"=w533:string)  [unwired: 12 in, 1 out]
        n221 = Enqueue Element(queue=w536, element=w533, error in (no error)=w535) -> (error out=w534:errorcluster)  [unwired: 1 in, 2 out]
      }
      event "Delete User": Value Change {
        # "sends deleteUser;/userName/password/type"
        # "deleteUser"
        n222 = event-data() -> ()  [unwired: 1 in, 1 out]
        n223 = local read "Edit username"() -> (w538:string)
        n224 = local read "Edit password"() -> (w537:string)
        n225 = local read "Type"() -> (w539:string)
        n226 = call "deleteUser"("userName"=w538, "password"=w537, "type"=w539) -> ("Result"=w540:string)  [unwired: 11 in, 1 out]
        n227 = Enqueue Element(queue=w543, element=w540, error in (no error)=w542) -> (error out=w541:errorcluster)  [unwired: 1 in, 2 out]
      }
      event "Product", "Quantity": Value Change {
        # "sends cost;Quantity/product"
        # "check if quantity change to get new cost"
        n228 = event-data() -> ()  [unwired: 1 in, 1 out]
        n229 = local read "Quantity"() -> (w544:dbl)
        n230 = local read "Product"() -> (w545:string)
        n231 = call "Cost"("Quantity"=w544, "product"=w545) -> ("Result"=w546:string)  [unwired: 12 in, 1 out]
        n232 = Enqueue Element(queue=w549, element=w546, error in (no error)=w548) -> (error out=w547:errorcluster)  [unwired: 1 in, 2 out]
      }
      event "stop": Value Change {
        # "Exit program execution"
        n233 = event-data() -> ()  [unwired: 1 in, 1 out]
      }
    }
    n234 = Unbundle By Name(w496) -> ("status"=w495:bool)
    n235 = Or(x=w495, y=w498) -> (x .or. y?=w497:bool)
  }
  n236 = Release Queue(queue=w1, error in (no error)=w7) -> ()  [unwired: 1 in, 3 out]
